vi "Transfer Group Error Info.vi"(11 "errors":T1) -> (3 "error info":cluster{"code":i32, "description":string})   [LabVIEW 2017, in "DSF Core.lvlib" / "Transfer Group.lvclass"]
uses:
  Transfer Group.lvclass
  Errors.ctl
  Framework/Base Error Code.vi
  Framework/Framework.lvclass
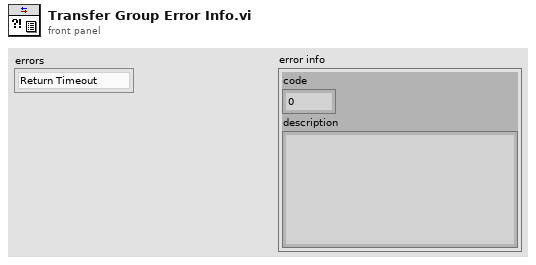
[diagram p1: front panel]
types:
  T1 = typedef "DSF Core.lvlib/Transfer Group.lvclass/Errors.ctl" = enum16{"Return Timeout", "Invalid Iteration"}
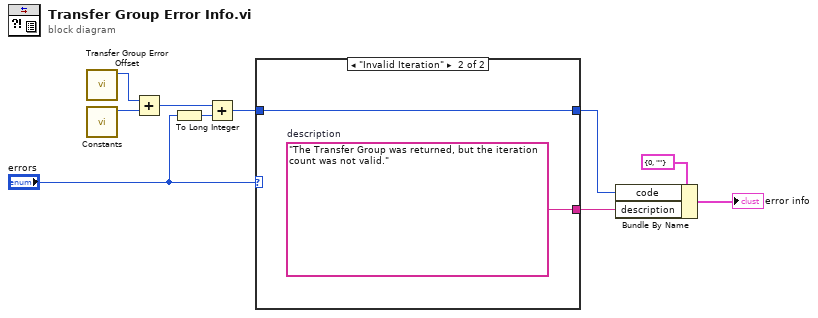
[diagram p0: block diagram]
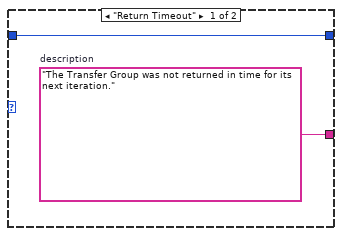
[diagram p2: hidden frame]
diagram:
  n1 = call "Transfer Group Error Offset.vi"() -> ("base error offset"=w2:i32)  [unwired: 11 in]
  n2 = call-poly "Constants.vi"() -> ("base error code"=w10:i32)  [unwired: 11 in]
  n3 = Add(x=w2, y=w10) -> (x+y=w6:i32)
  n4 = To Long Integer(number="errors") -> (32bit integer=w9:i32)
  n5 = Add(x=w6, y=w9) -> (x+y=w5:i32)
  n6 = case shown="\"Invalid Iteration\"" "errors" {
    tunnel: [w12 w14] -> w7
    tunnel: w5 -> [w11 w13]
    tunnel: [w11 w13] -> w4
    frame "Return Timeout" {
      w12 = "The Transfer Group was not returned in time for its next iteration."  # description
    }
    frame "Invalid Iteration" {
      w14 = "The Transfer Group was returned, but the iteration count was not valid."  # description
    }
  }
  n7 = Bundle By Name(cluster=cluster{"code":i32, "description":string} {"code"=0, "description"=""}, "code"=w4, "description"=w7) -> (→"error info":cluster{"code":i32, "description":string})
